vi "UT_005_LV to TOML.vi"() -> ()   [LabVIEW 2017]
uses:
  <vilib>/addons/_JKI Toolkits/Caraya/classes/Assert/Assert Error.vi
  <vilib>/addons/_JKI Toolkits/Caraya/classes/Test/Test.lvclass
  lib/TOML.lvlib
  <vilib>/addons/_JKI Toolkits/Caraya/classes/Assert/Assert.lvclass
panel:
  out "error out":errorcluster
  in  "data":string[][][](array[string])=[[["a", "b", "c"], ["d", "e", "f"], ["g", "h", "i"]]]
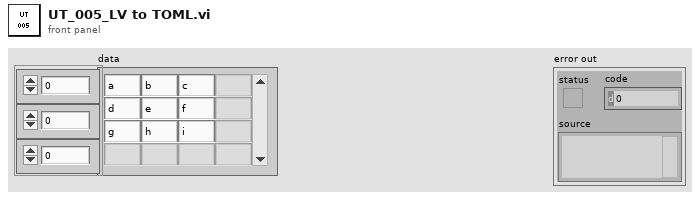
[diagram p1: front panel]
types:
  T1 = typedef "TOML.lvlib/TOML Value.ctl" = cluster{"type":enum16{"Table", "Array", "String", "Integer", "Float", "Boolean", "Offset Date-Time", "Local Date-Time", "Local Date", "Local Time", "Path"}, "value":variant}
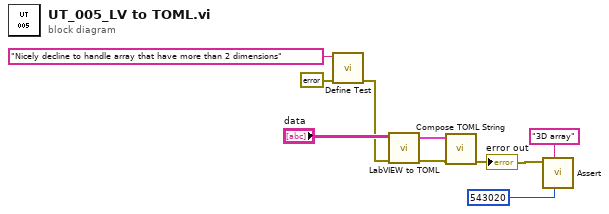
[diagram p0: block diagram]
diagram:
  n1 = call <vilib>:"Define Test.vi"("error in (no error)"=errorcluster {"status"=FALSE, "code"=0, "source"=""}, "Label (VI Title)"="Nicely decline to handle array that have more than 2 dimensions") -> ("error out"=w5:errorcluster)  [unwired: 9 in]
  n2 = call "LabVIEW to TOML.vi"("error in (no error)"=w5, "LV Value"="data") -> ("error out"=w3:errorcluster, "TOML Value"=w4:T1)  [unwired: 7 in, 1 out]
  n3 = call "Compose TOML String.vi"("error in (no error)"=w3, "Value"=w4) -> ("error out"=w1:errorcluster)  [unwired: 8 in, 1 out]
  "error out" <- w1
  n4 = call-poly <vilib>:"Assert.vi"("error code (1)"=543020, "Label"="3D array" ("Label (VI Title)"), "Error?"=w1) -> ()  [unwired: 8 in, 1 out]
